vi "OCV_Query.vi"(0 "System no.":i32=1 min=1 max=4 step=1, 2 "Axes to query":string[](array[string]), 5 "error in":errorcluster) -> (14 "Target position":dbl[](array[numeric]) format="%.6f", 19 "error out":errorcluster)   [LabVIEW 2020]
doc: "OCV? (Get Control Value)\n\nDescription\nQueries the current control value of the axes.\n\nFormat\nOCV?[ <AxisID>]\n\nArguments\nOCV? without arguments queries all axes of the controller.\n<AxisID>\nAn axis of the controller\nThe response to USG? CMD OCV? indicates in the #Related Units block for which axes the \ncommand can be used.\nPossible values: Alias of the axis (p. 94) \n\nResponse\n{<AxisID>\"=\"<ControlValue> LF}\n<ControlValue>\nCurrent control value\nThe unit used for the control value is dependent on the type of axis.\nThe data format is float.\nPossible values: Dependent on the type of axis\n\nExample\n>>eax?\n<<AXIS_1=1\n<<AXIS_2=1\n>>sam?\n<<AXIS_1=0x1\n<<AXIS_2=0x1\n>>pos?\n<<AXIS_1=136.0E-6 \n<<AXIS_2=-1.355E-3\n>>ocv axis_1 0.05\n>>ocv?\n<<AXIS_1=50.0E-3 \n<<AXIS_2=0\n>>ocv?\n<<AXIS_1=50.0E-3 \n<<AXIS_2=0\n>>pos?\n<<AXIS_1=13.490179\n<<AXIS_2=-1.405E-3\n>>err?\n<<0 - (error 0 - \"No error\")\n>>pos?\n<<AXIS_1=13.490194\n<<AXIS_2=-1.407E-3\n>>stp\n>>ocv?\n<<AXIS_1=0\n<<AXIS_2=0\n>>err?\n<<0 - (error 0 - \"No error\")\n>>stv?\n<<AXIS_1=0x1\n<<AXIS_2=0x1\n<<SYS_1=0x0\n>>log?\n<<#Error Information: <Index> <Timestamp> <Error Code>\n<Error Class> <Container Unit><Function Unit>\n<<1 74942661250 49159 CMD SYS_1 INTPR_3\n<<2 169045509375 81928 MOT SYS_1 INTPR_3 \n<<3 169046107500 81947 MOT AXIS_1 - \n<<4 169046110000 81947 MOT AXIS_2 - \n<<#END Error Information\n>>res axis_1\n>>stv?\n<<AXIS_1=0x0\n<<AXIS_2=0x1\n<<SYS_1=0x0\n>>res axis_2\n>>stv?\n<<AXIS_1=0x0\n<<AXIS_2=0x0\n<<SYS_1=0x0\n>>eax?\n<<AXIS_1=0\n<<AXIS_2=0\n>>sam?\n<<AXIS_1=0x0\n<<AXIS_2=0x0\n\nNotes\nThe parameter Axis_n - 0x109 Open-Loop Control Value shows the current control value. The \nvalue of this parameter can be read from the working memory of the controller using the SPV? \ncommand (p. 63); example for axis 1:\n>>spv? ram axis_1 - 0x109\n<<RAM AXIS_1 - 0x109=0.0\n\nUser command level\nUSR"
panel:
  # "OCV? (Get Control Value)\n\nQueries the current control value of the axes."
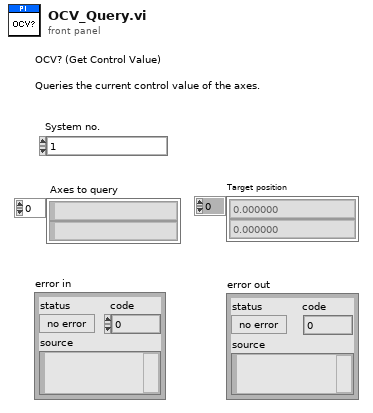
[diagram p1: front panel]
types:
  T1 = typedef "Syntax.ctl" = enum16{"GCS 1.0", "GCS 2.0", "GCS 3.0"}
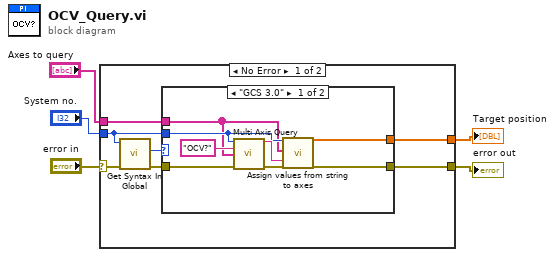
[diagram p0: block diagram]
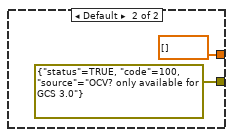
[diagram p2: hidden frame]
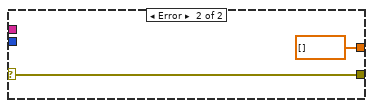
[diagram p3: hidden frame]
diagram:
  n1 = case shown="No Error" "error in" {
    selector: "error in" -> [w12 w24]
    tunnel: [w9 w24] -> w4
    tunnel: "Axes to query" -> [w8 _]
    tunnel: "System no." -> [w7 _]
    tunnel: [w6 dbl[] [] ("Target position")] -> w1
    frame No Error {
      n2 = call "Get Syntax In Global.vi"("error in"=w12, "System no."=w7) -> ("error out"=w10:errorcluster, "Syntax"=w11:T1)  [unwired: 8 in]
      n3 = case shown="\"GCS 3.0\"" w11 {
        tunnel: [w13 errorcluster {"status"=TRUE, "code"=100, "source"="OCV? only available for GCS 3.0"} ("error out")] -> w9
        tunnel: w10 -> [w17 _]
        tunnel: w8 -> [w15 _]
        tunnel: w7 -> [w16 _]
        tunnel: [w14 dbl[] [] ("Target position")] -> w6
        frame "GCS 3.0" {
          n4 = call "Multi Axis Query.vi"("System no."=w16, "Command"="OCV?", "Axis"=w15, "error in (no error)"=w17) -> ("Answer"=w19:string, "error out"=w20:errorcluster)  [unwired: 10 in]
          n5 = call "Assign values from string to axes.vi"("System no."=w16, "Queried axes"=w15, "Input String"=w19, "error in"=w20) -> ("Values"=w14:dbl[], "error out"=w13:errorcluster)  [unwired: 2 in, 12 out]
        }
        frame Default {
        }
      }
    }
    frame Error {
    }
  }
  "error out" <- w4
  "Target position" <- w1
